vi "Perform Step.vi"(8 "error in (no error)":errorcluster, 11 "Image Assertion in":refnum<class "Image Assertion.lvclass">) -> (0 "error out":errorcluster, 2 "Result":T1, 3 "Image Assertion out":refnum<class "Image Assertion.lvclass">)   [LabVIEW 2020, in "MacroAssert.lvlib" / "Image Assertion.lvclass"]
doc: "Performs all actions required for <B>Step in</B>."
uses:
  Image Assertion.lvclass
  C:/Users/User/Documents/LabVIEW Data/Projects/MacroAssert/source/Classes/Assertion Step/Assertion Step.lvclass
  Image Assertion.lvclass/Image Assertion.ctl
  MacroAssert.lvlib
  CTLs/Report Data.ctl
  SubVIs/Win Util/Win Util.lvlib
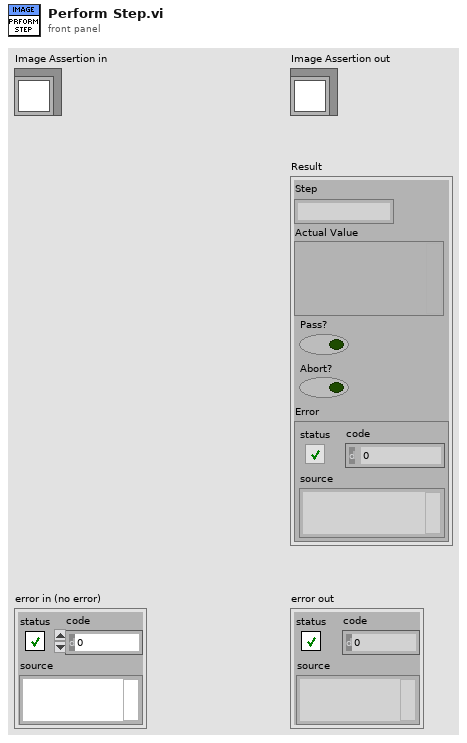
[diagram p1: front panel]
types:
  T1 = typedef "MacroAssert.lvlib/Report Data.ctl" = cluster{"Step":string, "Actual Value":variant, "Pass?":bool, "Abort?":bool, "Error":errorcluster}
  T2 = typedef "MacroAssert.lvlib/Image Assertion.lvclass/Image Comparator.ctl" = enum16{"Is less than or equal to", "Is greater than or equal to"}
  T3 = typedef "MacroAssert.lvlib/Image Assertion.lvclass/Compare Mode.ctl" = enum16{"Mean Squared Error", "Peak Signal-to-Noise Ratio"}
  T4 = typedef "imagedata.ctl" = cluster{"image type":i32, "image depth":i32, "image":u8[], "mask":u8[], "colors":u32[], "Rectangle":cluster{"left":i16, "top":i16, "right":i16, "bottom":i16}}
  T5 = typedef "MacroAssert.lvlib/Image Assertion.lvclass/Image Units.ctl" = enum16{"Pixels", "Percent"}
  T6 = typedef "MacroAssert.lvlib/Image Assertion.lvclass/Image Assertion Type.ctl" = enum16{"Control Image", "VI Image", "Window Image", "Cursor Icon"}
  T7 = typedef "MacroAssert.lvlib/Win Util.lvlib/Window Refnum.ctl" = u64
  T8 = cluster{"left":i16, "top":i16, "right":i16, "bottom":i16}
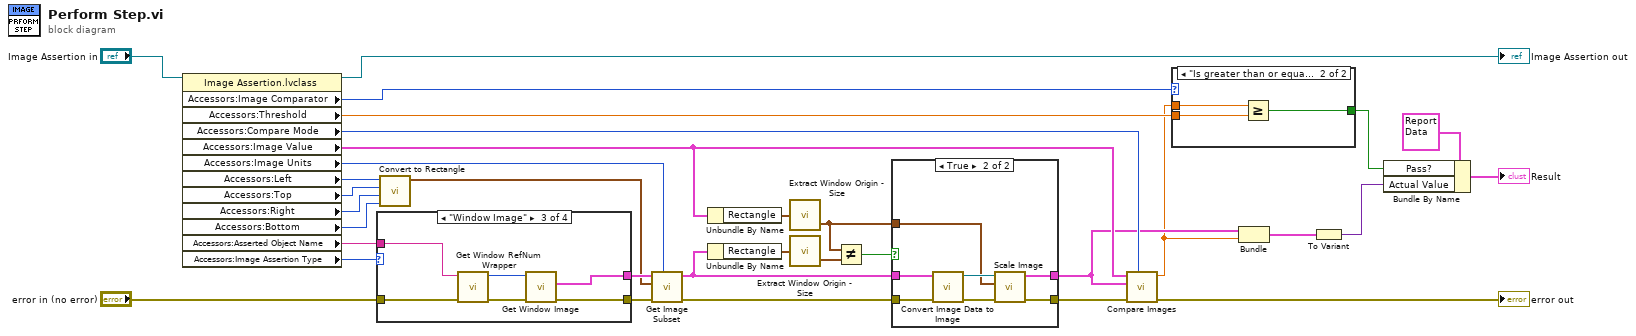
[diagram p0: block diagram]
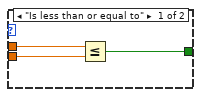
[diagram p3: hidden frame]
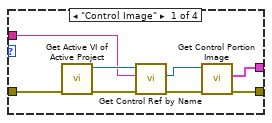
[diagram p4: hidden frame]
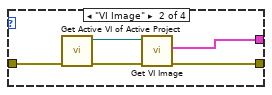
[diagram p5: hidden frame]
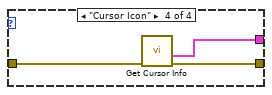
[diagram p6: hidden frame]
diagram:
  n1 = property class="Image Assertion.lvclass"(reference="Image Assertion in") -> (reference out=→"Image Assertion out":refnum<class "Image Assertion.lvclass">, "Accessors:Image Comparator"=w9:T2, "Accessors:Threshold"=w6:dbl, "Accessors:Compare Mode"=w8:T3, "Accessors:Image Value"=w11:T4, "Accessors:Image Units"=w18:T5, "Accessors:Left"=w25:i16, "Accessors:Top"=w24:i16, "Accessors:Right"=w23:i16, "Accessors:Bottom"=w22:i16, "Accessors:Asserted Object Name"=w26:string, "Accessors:Image Assertion Type"=w19:T6)  [unwired: 1 in, 1 out]
  n2 = case shown="\"Window Image\"" w19 {
    tunnel: "error in (no error)" -> [w37 w46 w51 w55]
    tunnel: [w36 w43 w52 w54] -> w21
    tunnel: [w35 w42 w48 w53] -> w20
    tunnel: w26 -> [w34 _ w47 _]
    frame "Control Image" {
      n3 = call "Get Active VI of Active Project.vi"("error in (no error)"=w37) -> ("error out"=w39:errorcluster, "Active VI Ref"=w38:refnum<vi>)  [unwired: 9 in]
      n4 = call "Get Control Ref by Name.vi"("error in (no error)"=w39, "Name"=w34, "VI Ref"=w38) -> ("error out"=w40:errorcluster, "Ctl Ref"=w41:refnum<vi>)  [unwired: 6 in, 1 out]
      n5 = call "Get Control Portion Image.vi"("error in (no error)"=w40, "Ctl Ref"=w41) -> ("error out"=w36:errorcluster, "Control Image"=w35:T4)  [unwired: 7 in, 1 out]
    }
    frame "VI Image" {
      n6 = call "Get Active VI of Active Project.vi"("error in (no error)"=w46) -> ("error out"=w45:errorcluster, "Active VI Ref"=w44:refnum<vi>)  [unwired: 9 in]
      n7 = call "Get VI Image.vi"("error in (no error)"=w45, "VI Ref"=w44) -> ("error out"=w43:errorcluster, "VI Image Data"=w42:T4)  [unwired: 7 in, 1 out]
    }
    frame "Window Image" {
      n8 = call "Get Window RefNum Wrapper.vi"("error in (no error)"=w51, "Window Name"=w47) -> ("error out"=w50:errorcluster, "window refnum"=w49:T7)  [unwired: 8 in]
      n9 = call "Get Window Image.vi"("error in (no error)"=w50, "window refnum in"=w49) -> ("error out"=w52:errorcluster, "image data"=w48:T4)  [unwired: 7 in, 1 out]
    }
    frame "Cursor Icon" {
      n10 = call "Get Cursor Info.vi"("error in (no error)"=w55) -> ("error out"=w54:errorcluster, "Image"=w53:T4)  [unwired: 6 in, 3 out]
    }
  }
  n11 = call "Convert to Rectangle.vi"("Bottom"=w22, "Right"=w23, "Top"=w24, "Left"=w25) -> ("Rectangle"=w16:T8)  [unwired: 7 in]
  n12 = call "Get Image Subset.vi"("Image Units"=w18, "error in (no error)"=w21, "Rectangle"=w16, "Image"=w20) -> ("error out"=w17:errorcluster, "Image Subset"=w5:T4)  [unwired: 6 in]
  n13 = Unbundle By Name(w11) -> ("Rectangle"=w15:T8)
  n14 = Unbundle By Name(w5) -> ("Rectangle"=w4:T8)
  n15 = call "Extract Window Origin - Size.vi"("window rect"=w15) -> ("window size"=w10:cluster{"Width":i16, "Height":i16})  [unwired: 1 out]
  n16 = call "Extract Window Origin - Size.vi"("window rect"=w4) -> ("window size"=w14:cluster{"Width":i16, "Height":i16})  [unwired: 1 out]
  n17 = Not Equal?(x=w10, y=w14) -> (x != y?=w12:bool)
  n18 = case shown="True" w12 {
    tunnel: w5 -> [w57 w64]
    tunnel: w17 -> [w56 w63]
    tunnel: [w56 w60] -> w13
    tunnel: [w57 w59] -> w2
    tunnel: w10 -> [_ w58]
    frame False {
    }
    frame True {
      n19 = call "Convert Image Data to Image.vi"("error in (no error)"=w63, "Image Data"=w64) -> ("error out"=w61:errorcluster, "Image Out"=w62:refnum<k24>)  [unwired: 8 in]
      n20 = call "Scale Image.vi"("error in (no error)"=w61, "New Dimensions"=w58, "Image"=w62) -> ("error out"=w60:errorcluster, "Scaled Image"=w59:T4)  [unwired: 7 in]
    }
  }
  n21 = call "Compare Images.vi"("Compare Mode"=w8, "error in (no error)"=w13, "Actual Image"=w2, "Expected Image"=w11) -> ("error out"=→"error out":errorcluster, "Value"=w1:dbl)  [unwired: 6 in]
  n22 = case shown="\"Is greater than or equal to\"" w9 {
    tunnel: [w67 w70] -> w28
    tunnel: w1 -> [w66 w69]
    tunnel: w6 -> [w65 w68]
    frame "Is less than or equal to" {
      n23 = Less Or Equal?(x=w66, y=w65) -> (x <= y?=w67:bool)
    }
    frame "Is greater than or equal to" {
      n24 = Greater Or Equal?(x=w69, y=w68) -> (x >= y?=w70:bool)
    }
  }
  n25 = Bundle("Scaled Image"=w2, "Value"=w1) -> (w3:cluster{"Scaled Image":T4, "Value":dbl})  [unwired: 1 in]
  n26 = To Variant(anything=w3) -> (Variant=w27:variant)
  n27 = Bundle By Name(cluster=T1 {"Step"="", "Actual Value"=variant, "Pass?"=FALSE, "Abort?"=FALSE, "Error"={"status"=FALSE, "code"=0, "source"=""}} ("Report Data"), "Pass?"=w28, "Actual Value"=w27) -> (→"Result":T1)
